vi "ErrorHandling.Filter.vi"(7 "source":string, 11 "remaining headers in":string) -> (3 "remaining headers out":string)   [LabVIEW 2013]
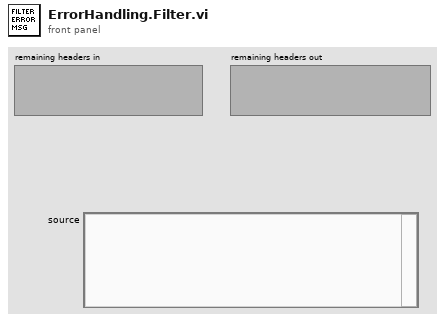
[diagram p1: front panel]
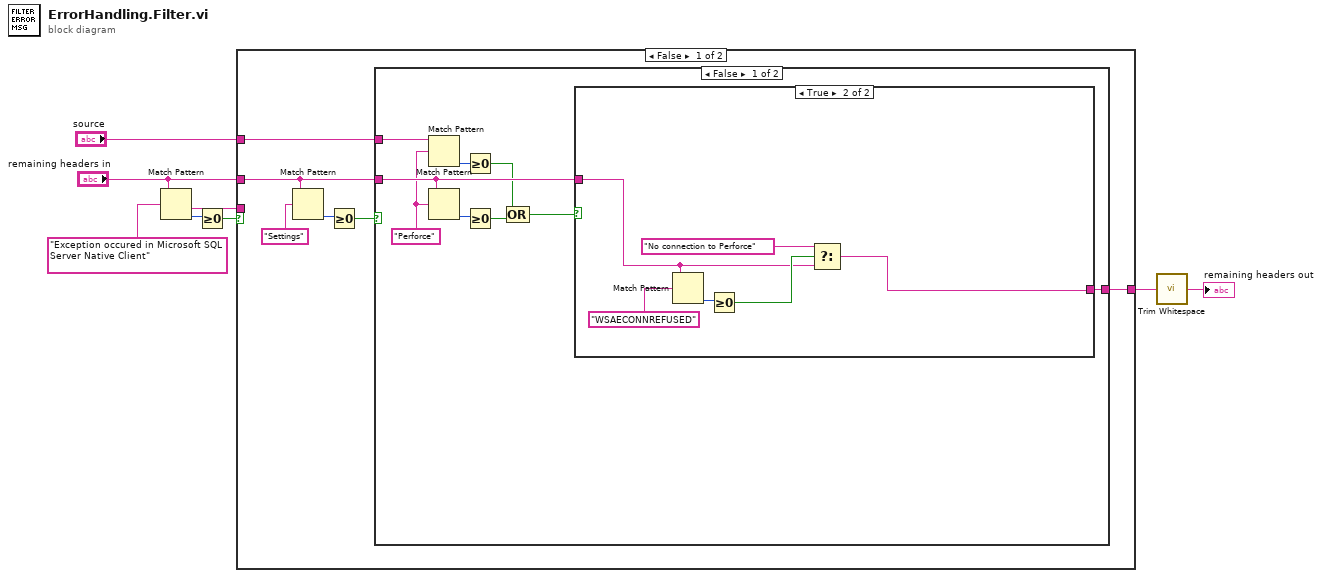
[diagram p0: block diagram]
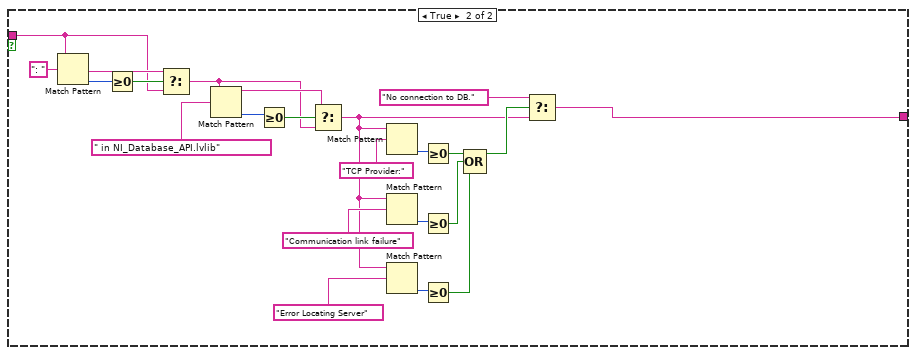
[diagram p4: hidden frame]
diagram:
  n1 = Match Pattern(string="remaining headers in", regular expression="Exception occured in Microsoft SQL Server Native Client") -> (after substring=w8:string, offset past match=w7:i32)  [unwired: 1 in, 2 out]
  n2 = Greater Or Equal To 0?(x=w7) -> (x >= 0?=w6:bool)
  n3 = case shown="False" w6 {
    tunnel: w8 -> [_ w45]
    tunnel: "remaining headers in" -> [w11 _]
    tunnel: [w10 w40] -> w4
    tunnel: "source" -> [w9 _]
    frame False {
      n4 = Match Pattern(string=w11, regular expression="Settings") -> (offset past match=w14:i32)  [unwired: 1 in, 3 out]
      n5 = Greater Or Equal To 0?(x=w14) -> (x >= 0?=w12:bool)
      n6 = case shown="False" w12 {
        tunnel: w11 -> [w21 w31]
        tunnel: [w22 w31] -> w10
        tunnel: w9 -> [w20 _]
        frame False {
          w19 = "Perforce" ("regular expression")
          n7 = Match Pattern(string=w20, regular expression=w19) -> (offset past match=w18:i32)  [unwired: 1 in, 3 out]
          n8 = Match Pattern(string=w21, regular expression=w19) -> (offset past match=w23:i32)  [unwired: 1 in, 3 out]
          n9 = Greater Or Equal To 0?(x=w18) -> (x >= 0?=w16:bool)
          n10 = Greater Or Equal To 0?(x=w23) -> (x >= 0?=w17:bool)
          n11 = Compound Arithmetic op=OR(w16, w17) -> (w15:bool)
          n12 = case shown="True" w15 {
            tunnel: [w24 w25] -> w22
            tunnel: w21 -> [w24 w26]
            frame False {
            }
            frame True {
              n13 = Match Pattern(string=w26, regular expression="WSAECONNREFUSED") -> (offset past match=w29:i32)  [unwired: 1 in, 3 out]
              n14 = Greater Or Equal To 0?(x=w29) -> (x >= 0?=w28:bool)
              n15 = Select(t="No connection to Perforce" ("regular expression"), s=w28, f=w26) -> (s? t:f=w25:string)
            }
          }
        }
        frame True {
        }
      }
    }
    frame True {
      n16 = Match Pattern(string=w45, regular expression=": ") -> (after substring=w47:string, offset past match=w48:i32)  [unwired: 1 in, 2 out]
      n17 = Greater Or Equal To 0?(x=w48) -> (x >= 0?=w49:bool)
      n18 = Select(t=w47, s=w49, f=w45) -> (s? t:f=w46:string)
      n19 = Match Pattern(string=w46, regular expression=" in NI_Database_API.lvlib") -> (before substring=w54:string, offset past match=w52:i32)  [unwired: 1 in, 2 out]
      n20 = Greater Or Equal To 0?(x=w52) -> (x >= 0?=w53:bool)
      n21 = Select(t=w54, s=w53, f=w46) -> (s? t:f=w34:string)
      n22 = Match Pattern(string=w34, regular expression="TCP Provider:") -> (offset past match=w43:i32)  [unwired: 1 in, 3 out]
      n23 = Match Pattern(string=w34, regular expression="Communication link failure") -> (offset past match=w39:i32)  [unwired: 1 in, 3 out]
      n24 = Match Pattern(string=w34, regular expression="Error Locating Server") -> (offset past match=w35:i32)  [unwired: 1 in, 3 out]
      n25 = Greater Or Equal To 0?(x=w43) -> (x >= 0?=w42:bool)
      n26 = Greater Or Equal To 0?(x=w39) -> (x >= 0?=w33:bool)
      n27 = Greater Or Equal To 0?(x=w35) -> (x >= 0?=w32:bool)
      n28 = Compound Arithmetic op=OR(w42, w33, w32) -> (w37:bool)
      n29 = Select(t="No connection to DB." ("regular expression"), s=w37, f=w34) -> (s? t:f=w40:string)
    }
  }
  n30 = call <vilib>:"Trim Whitespace.vi"("string"=w4) -> ("trimmed string"=→"remaining headers out":string)  [unwired: 1 in]
